vi "destroy.vi"(8 "error in":errorcluster, 11 "close reference and report in":refnum<class "close reference and report.lvclass">) -> (0 "error out":errorcluster)   [LabVIEW 2013, in "close reference and report.lvclass"]
uses:
  close reference and report.lvclass
  close reference and report.lvclass/close reference and report.ctl
  results reporter/results reporter.lvclass
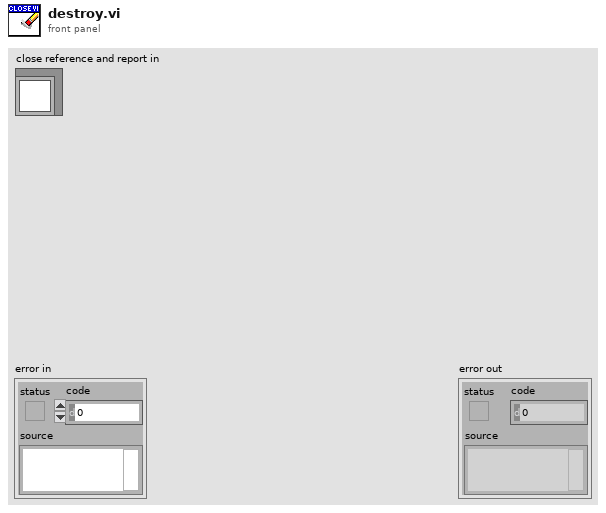
[diagram p1: front panel]
types:
  T1 = typedef "call by reference action.lvclass/function definition.ctl" = refnum<vi>
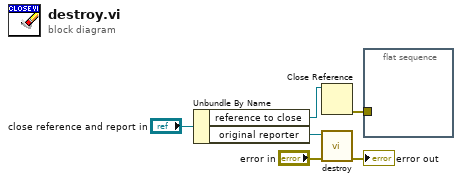
[diagram p0: block diagram]
diagram:
  n1 = Unbundle By Name("close reference and report in") -> ("reference to close"=w2:T1, "original reporter"=w5:refnum<class "results reporter.lvclass">)
  n2 = Close Reference(reference=w2) -> (error out=w1:errorcluster)  [unwired: 1 in]
  n3 = call-dynamic "destroy.vi"("error in"="error in", "results reporter in"=w5) -> ("error out"=→"error out":errorcluster)  [unwired: 9 in]
  n4 = flat-sequence {
    tunnel: w1 -> [_]
    frame #0 {
    }
  }
